vi "Display.vi"(8 "Error In":errorcluster, 11 "Error-Prompt in":refnum<class "Error-Prompt.lvclass">) -> (0 "Error Out":errorcluster, 3 "Error-Prompt out":refnum<class "Error-Prompt.lvclass">)   [LabVIEW 2021, in "Pop-Up.lvlib" / "Error-Prompt.lvclass"]
doc: "Display method for an error prompt\n\n<b>Code Developed By:</b> +\nDaniel Coons +\nhttps://github.com/danielcoons/tsc-pop-up"
uses:
  Error-Prompt.lvclass
  C:/Development/Open Source/tsc-pop-up/Popup/Popup.lvclass
  Popup/Popup.lvclass/Popup.ctl
  Theme/Theme.lvclass/Theme.ctl
  Theme/Theme.lvclass
  Error-Prompt.lvclass/Error-Prompt.ctl
  Popup/Popup.lvclass
  user32.dll
panel:
  in  "n-choice":bool
  in  "y-choice":bool
  out "header":bool
  out "Message":string
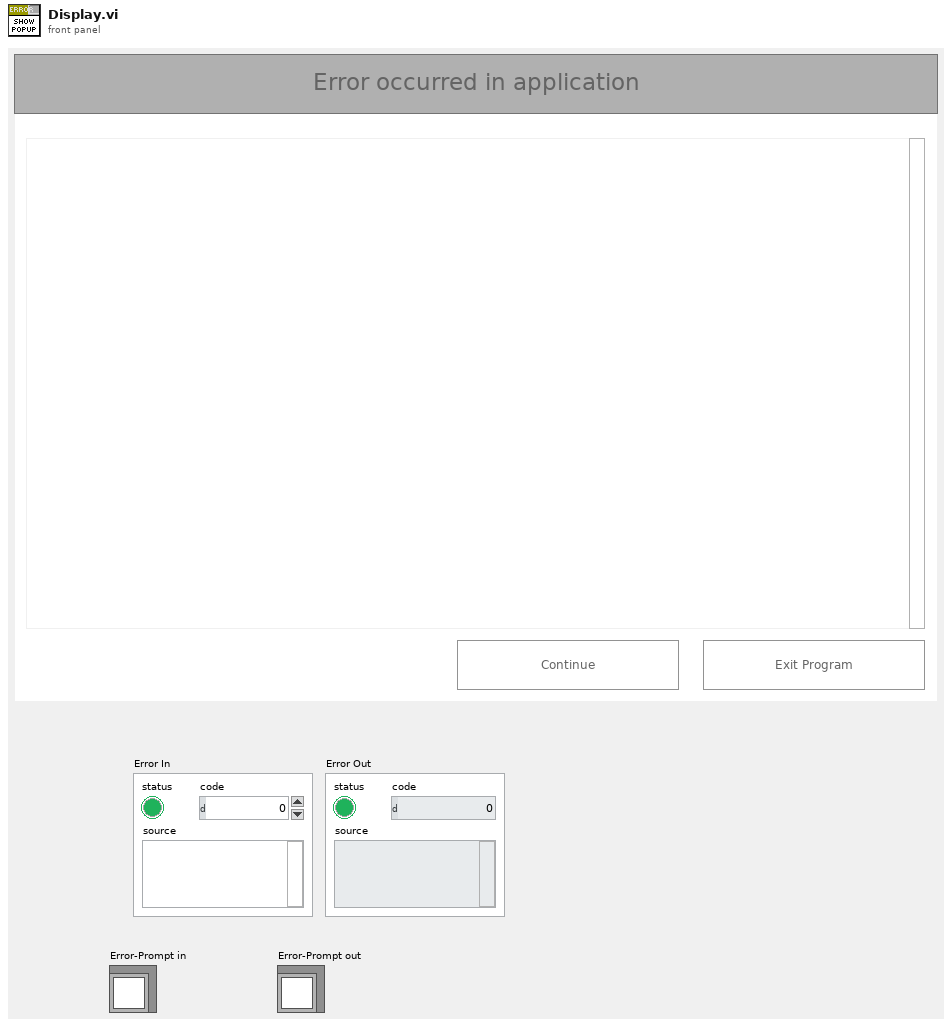
[diagram p1: front panel]
types:
  T1 = typedef "Theme.lvclass/message box--typdef.ctl" = cluster{"Text.Font Name":string, "Text.Font Size":u32, "Color":u32, "Text.Justification":enum16{"Left", "Center", "Right"}, "messge color":cluster{"border":u32, "fill":u32}}
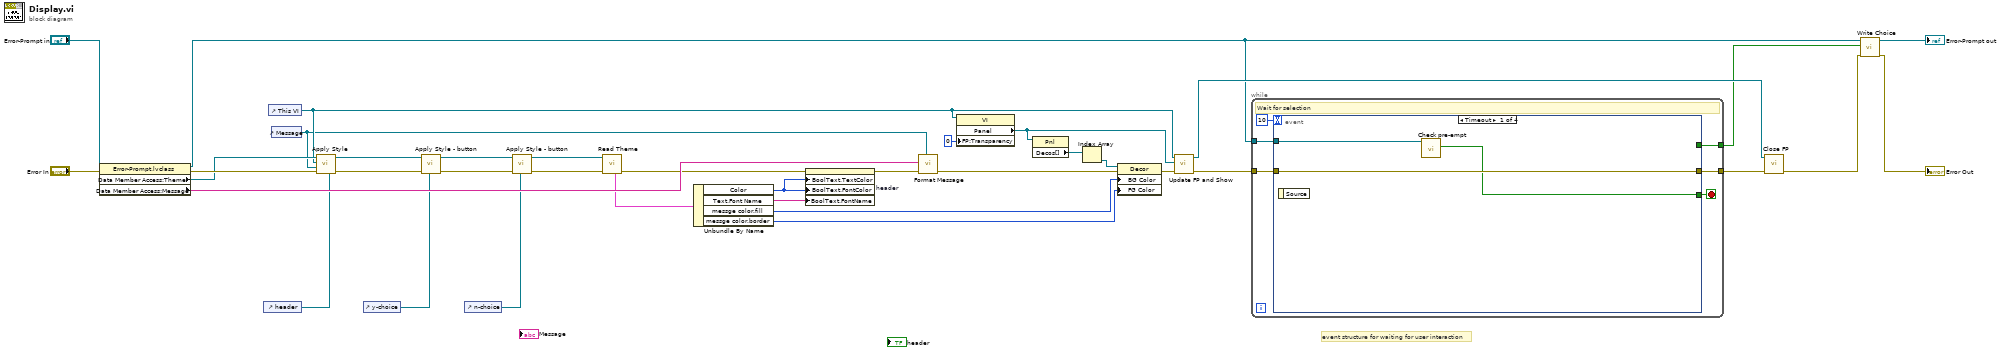
[diagram p0: block diagram]
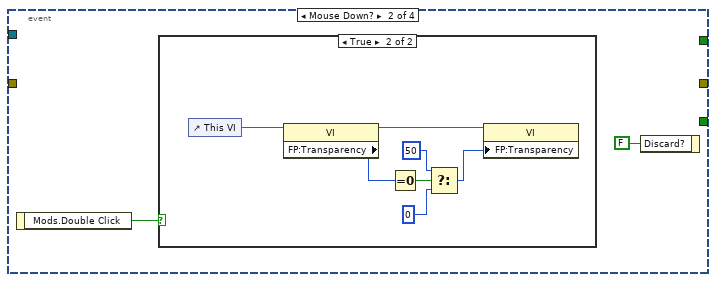
[diagram p2: hidden frame]
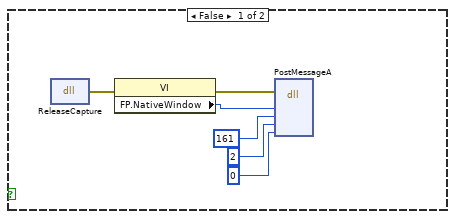
[diagram p3: hidden frame]
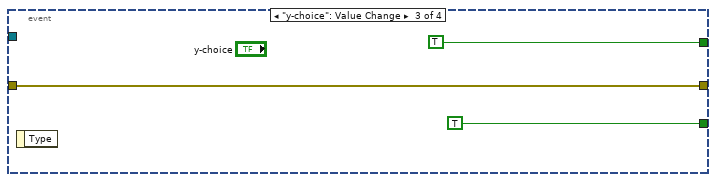
[diagram p4: hidden frame]
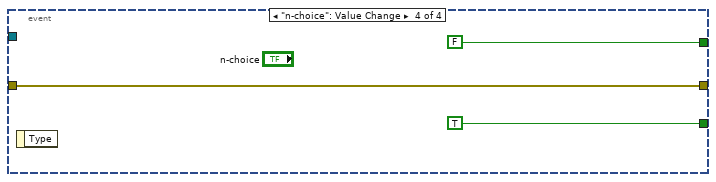
[diagram p5: hidden frame]
diagram:
  # "event structure for waiting for user interaction"
  n1 = property class="Error-Prompt.lvclass"(reference="Error-Prompt in", error in="Error In") -> (reference out=w25:refnum<class "Error-Prompt.lvclass">, error out=w37:errorcluster, "Data Member Access:Theme"=w30:refnum<class "Theme.lvclass">, "Data Member Access:Message"=w33:string)
  n2 = control-ref of="header"() -> (w27:refnum<vi>)
  n3 = control-ref of="This VI"() -> (w29:refnum<vi>)
  n4 = control-ref of="Message"() -> (w28:refnum<vi>)
  n5 = call "Apply Style.vi"("header ref"=w27, "error in"=w37, "message ref"=w28, "pop up ref"=w29, "Theme in"=w30) -> ("error out"=w31:errorcluster, "Theme out"=w21:refnum<class "Theme.lvclass">)  [unwired: 5 in]
  n6 = control-ref of="y-choice"() -> (w20:refnum<vi>)
  n7 = call "Apply Style - button.vi"("button ref"=w20, "error in"=w31, "Theme in"=w21) -> ("error out"=w22:errorcluster, "Theme out"=w19:refnum<class "Theme.lvclass">)  [unwired: 7 in]
  n8 = control-ref of="n-choice"() -> (w18:refnum<vi>)
  n9 = call "Apply Style - button.vi"("button ref"=w18, "error in"=w22, "Theme in"=w19) -> ("error out"=w23:errorcluster, "Theme out"=w13:refnum<class "Theme.lvclass">)  [unwired: 7 in]
  n10 = call "Read Theme.vi"("error in"=w23, "Theme in"=w13) -> ("error out"=w6:errorcluster, "message font"=w2:T1)  [unwired: 5 in, 3 out]
  n11 = Unbundle By Name(w2) -> ("Color"=w3:u32, "Text.Font Name"=w4:string, "messge color.fill"=w8:u32, "messge color.border"=w7:u32)
  n12 = property on="header" class="Bool (strict)"(error in=w6, "BoolText.TextColor"=w3, "BoolText.FontColor"=w3, "BoolText.FontName"=w4) -> (error out=w5:errorcluster)  [unwired: 1 in, 1 out]
  n13 = call "Format Message.vi"("formatted string"=w28, "error in"=w5, "String Input"=w33) -> ("error out"=w32:errorcluster)  [unwired: 7 in, 1 out]
  n14 = property class="VI"(reference=w29, "FP:Transparency"=u8 0 ("Front Panel Window:Transparency")) -> ("Panel"=w12:refnum<vi>)  [unwired: 1 in, 2 out]
  n15 = property class="Pnl"(reference=w12) -> ("Decos[]"=w11:refnum<vi>[])  [unwired: 1 in, 2 out]
  n16 = Index Array(array=w11) -> (element=w9:refnum<vi>)  [unwired: 1 in]
  n17 = property class="Decor"(reference=w9, error in=w32, "BG Color"=w8, "FG Color"=w7) -> (error out=w10:errorcluster)  [unwired: 1 out]
  n18 = call "Update FP and Show.vi"("error in (no error)"=w10, "Panel Ref"=w12, "VI in"=w29) -> ("error out"=w35:errorcluster, "VI out"=w34:refnum<vi>)  [unwired: 7 in]
  n19 = while {
    tunnel: [w41] -> w36
    tunnel: w35 -> [w42]
    tunnel: w25 -> [w39]
    tunnel: [w38] -> w14
    stop <- w43 stop-if-true
    # "Wait for selection"
    n20 = event shown="[0] Timeout" {
      selector: _ -> [_ _ _ _]
      dyn-events: _ -> [_ _ _ _]
      timeout: 10 -> [_ _ _ _]
      tunnel: [w44 _ TRUE ("Pre-empted?") TRUE ("Pre-empted?")] -> w43
      tunnel: w42 -> [w46 _ w63 w66]
      tunnel: [w46 _ w63 w66] -> w41
      tunnel: w39 -> [w45 _ _ _]
      tunnel: [_ _ TRUE FALSE] -> w38
      event Timeout {
        n21 = event-data() -> ()  [unwired: 1 in, 1 out]
        n22 = call "Check pre-empt.vi"("_Popup in"=w45) -> ("Pre-empted?"=w44:bool)  [unwired: 8 in, 2 out]
      }
      event Mouse Down? {
        n23 = event-data() -> ("Mods.Double Click"=w47:bool)  [unwired: 1 in]
        n24 = case shown="True" w47 {
          frame False {
            n25 = dll-call lib="user32.dll" fn="ReleaseCapture"() -> (error out=w52:errorcluster)  [unwired: 4 in, 1 out]
            n26 = property class="VI"(error in=w52) -> (error out=w53:errorcluster, "FP.NativeWindow"=w54:u64)  [unwired: 1 in, 1 out]
            n27 = dll-call lib="user32.dll" fn="PostMessageA"(error in=w53, "hWnd"=w54, "Msg"=161, "wParam"=2, "lParam"=0) -> ()  [unwired: 7 in, 2 out]
          }
          frame True {
            n28 = control-ref of="This VI"() -> (w61:refnum<vi>)
            n29 = property class="VI"(reference=w61) -> (reference out=w59:refnum<vi>, "FP:Transparency"=w60:u8)  [unwired: 1 in, 1 out]
            n30 = Equal To 0?(x=w60) -> (x = 0?=w58:bool)
            n31 = Select(t=u8 50, s=w58, f=u8 0) -> (s? t:f=w55:u8)
            n32 = property class="VI"(reference=w59, "FP:Transparency"=w55) -> ()  [unwired: 1 in, 2 out]
          }
        }
        n33 = event-data("Discard?"=FALSE) -> ()  [unwired: 1 in, 1 out]
      }
      event "y-choice": Value Change {
        n34 = event-data() -> ()  [unwired: 1 in, 1 out]
      }
      event "n-choice": Value Change {
        n35 = event-data() -> ()  [unwired: 1 in, 1 out]
      }
    }
  }
  n36 = call "Close FP.vi"("error in (no error)"=w36, "VI in"=w34) -> ("error out"=w16:errorcluster)  [unwired: 9 in]
  n37 = call-dynamic "Write Choice.vi"("error in (no error)"=w16, "Choice"=w14, "_Popup in"=w25) -> ("error out"=→"Error Out":errorcluster, "_Popup out"=→"Error-Prompt out":refnum<class "Error-Prompt.lvclass">)  [unwired: 7 in]
